vi "Read Port.vi"(8 "error in (no error)":errorcluster, 9 "Port 2":u16, 10 "VISA resource name":refnum<visa-resource-name>, 11 "Cypress in":refnum<class "Cypress.lvclass">) -> (0 "error out":errorcluster, 1 "String":string, 2 "VISA resource name 2":refnum<visa-resource-name>, 3 "Cypress out":refnum<class "Cypress.lvclass">)   [LabVIEW 2020, in "Cypress.lvclass"]
uses:
  Cypress.lvclass
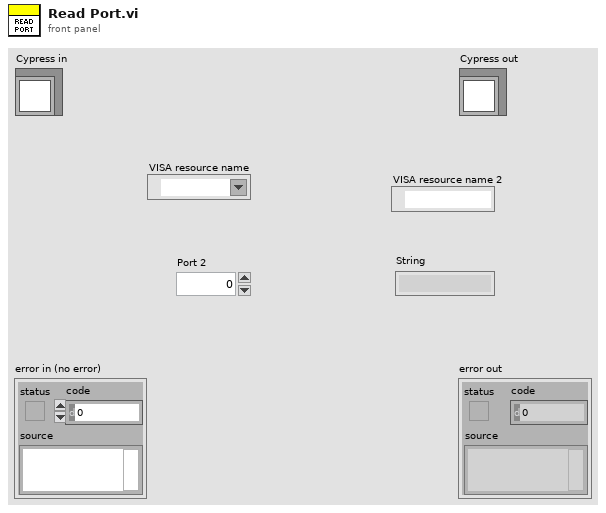
[diagram p1: front panel]
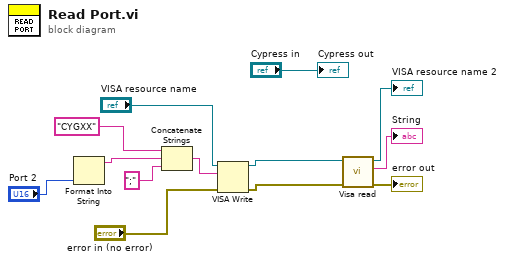
[diagram p0: block diagram]
diagram:
  n1 = Format Into String("Port 2") -> (resulting string=w2:string)  [unwired: 3 in, 1 out]
  n2 = Concatenate Strings("CYGXX" ("string"), w2, ";" ("string")) -> (w4:string)
  n3 = VISA Write(VISA resource name="VISA resource name", write buffer=w4, error in (no error)="error in (no error)") -> (VISA resource name out=w7:refnum<visa-resource-name>, error out=w6:errorcluster)  [unwired: 1 out]
  n4 = call "Visa read.vi"("error in (no error)"=w6, "VISA Refnum in"=w7) -> ("error out"=→"error out":errorcluster, "String"=→"String":string, "VISA Refnum out"=→"VISA resource name 2":refnum<visa-resource-name>)  [unwired: 7 in]
  "Cypress out" <- "Cypress in"
